vi "Arm State Machine.vi"(6 "Reset":bool, 7 "Tote Count":dbl format="%#_13g", 8 "Emergency Release":bool, 10 "Claw":bool=TRUE, 11 "Arm Button":bool=TRUE) -> ()   [LabVIEW 2014]
uses:
  TypeDefs/SRE Enum.ctl
  Support Code/Robot Global Data.vi
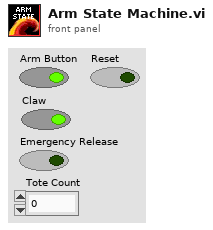
[diagram p1: front panel]
types:
  T1 = enum16{"Arm Down Open", "Arm Down Closed", "Arm Mid", "Arm Release", "Arm Up"}
  T2 = typedef "SRE Enum.ctl" = enum16{"Start", "Run", "End"}
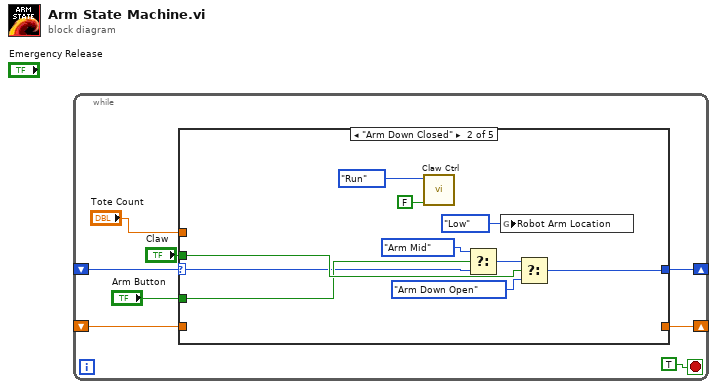
[diagram p0: block diagram]
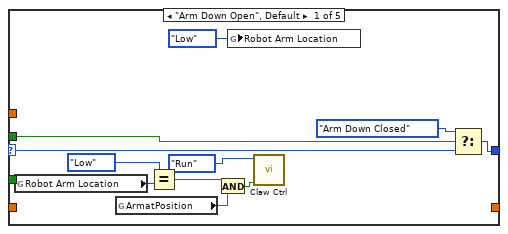
[diagram p2: hidden frame]
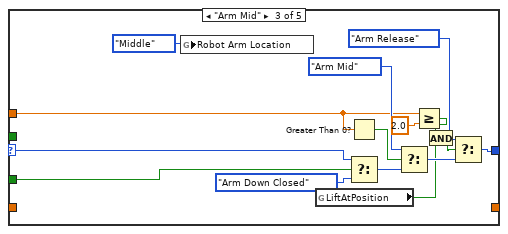
[diagram p3: hidden frame]
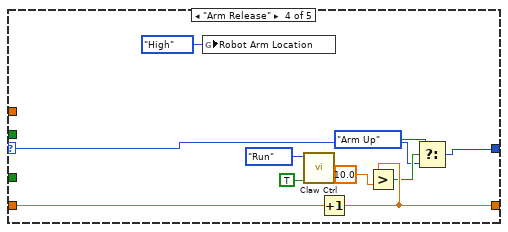
[diagram p4: hidden frame]
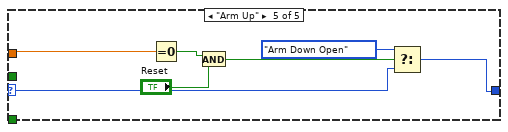
[diagram p5: hidden frame]
diagram:
  n1 = while {
    shift-right: [w6] -> _
    shift-left: _ -> [w7]
    shift-right: [w3] -> _
    shift-left: _ -> [w2]
    stop <- TRUE stop-if-true
    n2 = case shown="\"Arm Down Closed\"" w7 {
      selector: w7 -> [w17 w22 w39 w47 w57]
      tunnel: [w15 w26 w35 w45 w58] -> w6
      tunnel: "Claw" -> [w14 w27 _ _ _]
      tunnel: "Arm Button" -> [_ w24 w44 _ _]
      tunnel: [_ _ _ w49 _] -> w3
      tunnel: w2 -> [_ _ _ w51 _]
      tunnel: "Tote Count" -> [_ _ w33 _ w61]
      frame "Arm Down Open", Default {
        n3 = global read "Robot Global Data.vi" "Robot Arm Location"() -> (w11:enum16{"High", "Middle", "Low"})
        n4 = global read "Robot Global Data.vi" "ArmatPosition"() -> (w13:bool)
        n5 = Equal?(x=enum16{"High", "Middle", "Low"}."Low", y=w11) -> (x = y?=w9:bool)
        n6 = And(x=w9, y=w13) -> (x .and. y?=w12:bool)
        n7 = global write "Robot Global Data.vi" "Robot Arm Location"(enum16{"High", "Middle", "Low"}."Low" ("Robot Arm Location")) -> ()
        n8 = call "Claw Ctrl.vi"("Open/Close"=w12, "Enum"=SRE_Enum."Run") -> ()  [unwired: 10 in]
        n9 = Select(t=T1."Arm Down Closed", s=w14, f=w17) -> (s? t:f=w15:T1)
      }
      frame "Arm Down Closed" {
        n10 = call "Claw Ctrl.vi"("Open/Close"=FALSE, "Enum"=SRE_Enum."Run") -> ()  [unwired: 10 in]
        n11 = Select(t=T1."Arm Mid", s=w24, f=w22) -> (s? t:f=w23:T1)
        n12 = global write "Robot Global Data.vi" "Robot Arm Location"(enum16{"High", "Middle", "Low"}."Low" ("Robot Arm Location")) -> ()
        n13 = Select(t=w23, s=w27, f=T1."Arm Down Open" ("Arm State")) -> (s? t:f=w26:T1)
      }
      frame "Arm Mid" {
        n14 = global write "Robot Global Data.vi" "Robot Arm Location"(enum16{"High", "Middle", "Low"}."Middle" ("Robot Arm Location")) -> ()
        n15 = global read "Robot Global Data.vi" "LiftAtPosition"() -> (w31:bool)
        n16 = Greater Than 0?(x=w33) -> (x > 0?=w42:bool)
        n17 = Select(t=w39, s=w44, f=T1."Arm Down Closed" ("Arm State")) -> (s? t:f=w41:T1)
        n18 = Select(t=T1."Arm Mid", s=w42, f=w41) -> (s? t:f=w38:T1)
        n19 = Greater Or Equal?(x=w33, y=2.0) -> (x >= y?=w32:bool)
        n20 = And(x=w32, y=w31) -> (x .and. y?=w30:bool)
        n21 = Select(t=T1."Arm Release", s=w30, f=w38) -> (s? t:f=w35:T1)
      }
      frame "Arm Release" {
        n22 = global write "Robot Global Data.vi" "Robot Arm Location"(enum16{"High", "Middle", "Low"}."High" ("Robot Arm Location")) -> ()
        n23 = call "Claw Ctrl.vi"("Open/Close"=TRUE, "Enum"=SRE_Enum."Run") -> ()  [unwired: 10 in]
        n24 = Increment(x=w51) -> (x+1=w49:dbl)
        n25 = Greater?(x=w49, y=10.0 ("x")) -> (0:w48:bool)
        n26 = Select(t=T1."Arm Up", s=w48, f=w47) -> (s? t:f=w45:T1)
      }
      frame "Arm Up" {
        n27 = Equal To 0?(x=w61) -> (x = 0?=w60:bool)
        n28 = And(x=w60, y="Reset") -> (x .and. y?=w59:bool)
        n29 = Select(t=T1."Arm Down Open", s=w59, f=w57) -> (s? t:f=w58:T1)
      }
    }
  }
